vi "Transceiver Thread.Get Transceiver.vi"(11 "Transceiver Thread in":refnum<class "Transceiver Thread.lvclass">) -> (2 "Transceiver":refnum<class "Transceiver.lvclass">, 3 "Transceiver Thread out":refnum<class "Transceiver Thread.lvclass">)   [LabVIEW 2017, in "DSF.Engine.lvlib" / "Transceiver Thread.lvclass"]
uses:
  Transceiver Thread.lvclass
  Transceiver.lvclass
  Transceiver Thread.lvclass/Transceiver Thread.ctl
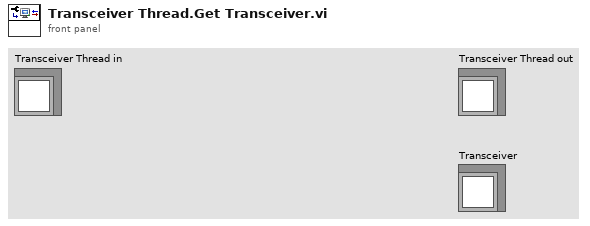
[diagram p1: front panel]
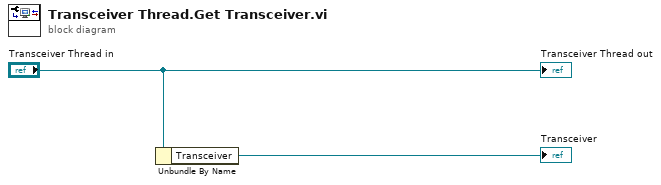
[diagram p0: block diagram]
diagram:
  n1 = Unbundle By Name("Transceiver Thread in") -> ("Transceiver"=→"Transceiver":refnum<class "Transceiver.lvclass">)
  "Transceiver Thread out" <- "Transceiver Thread in"
